vi "RTT_ZC_Method (SubVI).vi"(10 "P BWD":waveform(dbl), 11 "P FWD":waveform(dbl)) -> (3 "RTT (ms)":dbl)   [LabVIEW 2017]
uses:
  <vilib>/Analysis/NI_AALBase.lvlib
  <vilib>/Analysis/baseanly.llb/Mean (DBL).vi
panel:
  out "Waveform Graph":dbl[][](graph)
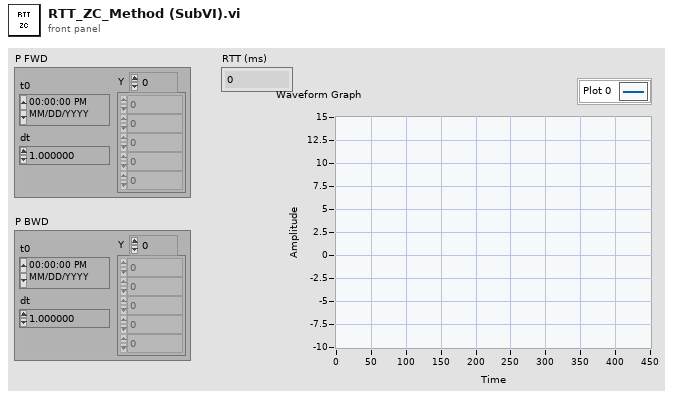
[diagram p1: front panel]
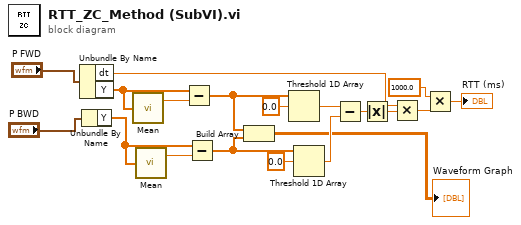
[diagram p0: block diagram]
diagram:
  n1 = Unbundle By Name("P FWD") -> ("dt"=w14:dbl, "Y"=w4:dbl[])
  n2 = Unbundle By Name("P BWD") -> ("Y"=w7:dbl[])
  n3 = call-poly <vilib>:"Mean.vi"("X"=w4) -> ("mean"=w5:dbl)  [unwired: 1 out]
  n4 = call-poly <vilib>:"Mean.vi"("X"=w7) -> ("mean"=w6:dbl)  [unwired: 1 out]
  n5 = Subtract(x=w4, y=w5) -> (x-y=w8:dbl[])
  n6 = Subtract(x=w7, y=w6) -> (x-y=w11:dbl[])
  n7 = Build Array(w8, w11) -> (→"Waveform Graph":dbl[][])
  n8 = Threshold 1D Array(2:0.0 ("threshold y"), 3:w8) -> (0:w12:dbl)  [unwired: 1 in]
  n9 = Threshold 1D Array(2:0.0 ("threshold y"), 3:w11) -> (0:w13:dbl)  [unwired: 1 in]
  n10 = Subtract(x=w12, y=w13) -> (x-y=w18:dbl)
  n11 = Absolute Value(x=w18) -> (abs(x)=w19:dbl)
  n12 = Multiply(x=w14, y=w19) -> (x*y=w15:dbl)
  n13 = Multiply(x=1000.0 ("threshold y"), y=w15) -> (x*y=→"RTT (ms)":dbl)
